vi "On Connect.vi"(8 "error in (no error)":errorcluster, 10 "Actor in":refnum<class "Actor.lvclass">, 11 "Client Connection Handler Msg in":refnum<class "Client Connection Handler Msg.lvclass">) -> (0 "error out":errorcluster, 2 "Actor out":refnum<class "Actor.lvclass">, 3 "Client Connection Handler Msg out":refnum<class "Client Connection Handler Msg.lvclass">)   [LabVIEW 2021, in "Secure Echo Broadcast With Server Manager.lvlib" / "Client Connection Handler Msg.lvclass"]
uses:
  Client Connection Handler Msg.lvclass
  C:/Projects/WebSocket-Actor/WebSocket Actor/Abstract Messages/WebSocket Connection Handler Msg/WebSocket Connection Handler Msg.lvclass
  <vilib>/ActorFramework/Actor/Actor.lvclass
  WS Client Subscriber/WS Client Subscriber.lvclass
  C:/Program Files/National Instruments/LabVIEW 2021/vi.lib/ActorFramework/Actor/Actor.lvclass
  WebSocket Actor/Abstract Messages/WebSocket Connection Handler Msg/WebSocket Connection Handler Msg.lvclass/WebSocket Connection Handler Msg.ctl
  WebSocket Actor/Abstract Messages/WebSocket Connection Handler Msg/properties/Read Connection Enqueuer.vi
  <vilib>/ActorFramework/Message Enqueuer/Message Enqueuer.lvclass
  Client Connection Handler Msg.lvclass/Client Connection Handler Msg.ctl
  C:/Projects/WebSocket-Actor/Examples/Secure Echo Broadcast With Server Manager/WS Client Subscriber/WS Client Subscriber.lvclass
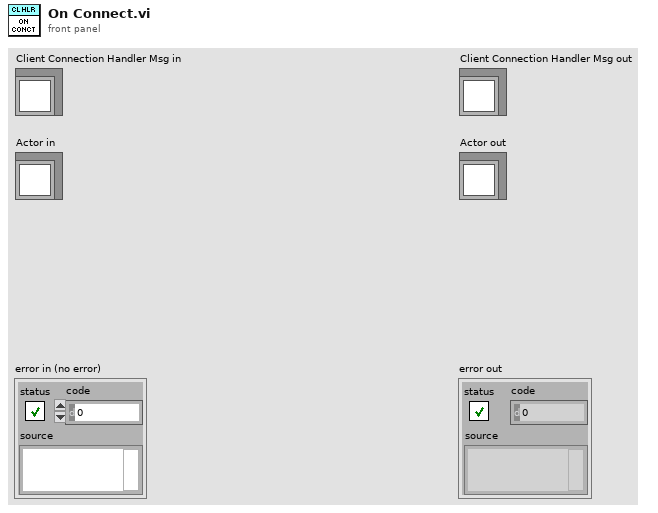
[diagram p1: front panel]
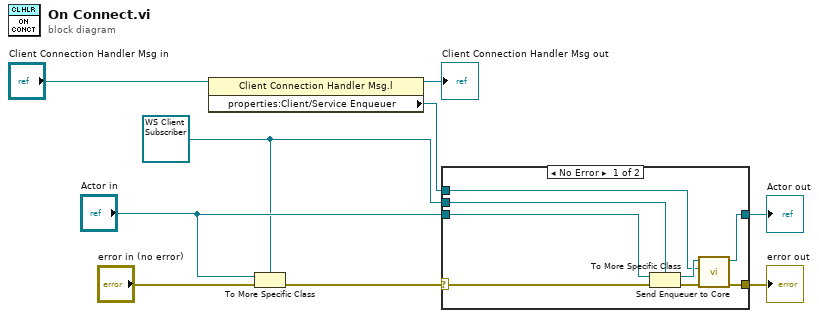
[diagram p0: block diagram]
diagram:
  w5 = refnum<class "WS Client Subscriber.lvclass"> refnum ("WS Full LabVIEW Test.lvlib:WS Test Client.lvclass")
  n1 = property class="Client Connection Handler Msg.l"(reference="Client Connection Handler Msg in") -> (reference out=→"Client Connection Handler Msg out":refnum<class "Client Connection Handler Msg.lvclass">, "properties:Client/Service Enqueuer"=w3:refnum<class "Message Enqueuer.lvclass">)  [unwired: 1 in, 1 out]
  n2 = To More Specific Class(target class=w5, reference="Actor in", error in="error in (no error)") -> (error out=w7:errorcluster)  [unwired: 1 out]
  n3 = case shown="No Error" w7 {
    selector: w7 -> [w15 w18]
    tunnel: "Actor in" -> [w17 w19]
    tunnel: w5 -> [w16 _]
    tunnel: w3 -> [w12 _]
    tunnel: [w11 w18] -> w2
    tunnel: [w10 w19] -> w1
    frame No Error {
      n4 = To More Specific Class(target class=w16, reference=w17, error in=w15) -> (specific class reference=w13:refnum<class "WS Client Subscriber.lvclass">, error out=w14:errorcluster)
      n5 = call "Send Enqueuer to Core.vi"("error in (no error)"=w14, "Client/Service Enqueuer"=w12, "WS Test Client in"=w13) -> ("error out"=w11:errorcluster, "WS Test Client out"=w10:refnum<class "WS Client Subscriber.lvclass">)  [unwired: 7 in]
    }
    frame Error {
    }
  }
  "error out" <- w2
  "Actor out" <- w1
